vi "decode-from-json-cDAQ.vi"(8 "sensor-options-json":string, 10 "data-logging-json":string, 11 "filepath-json":string) -> (0 "Sensor Option Recall":T1={"Display Units"="log", "Zero Offset"=2.62, "Sensor Min"=0.0, "Sensor Max"=500.0, "Signal Min"=0.0, "Signal Max"=100.0, "Conversion Factor"=0.0}, 2 "Datalogging Recall":T2={"data-precision"=3, "Include Date"=FALSE, "Include Timestamp"=TRUE, "Include Milliseconds"=FALSE, "sample-rate (Hz)"=4.0, "Logging Active"=TRUE}, 3 "Filepath Recall":T3={"Log Filepath Source"=enum."Application Relative (Auto)", "Log File Path (Manual)"=path "C:/Users/dheard/Documents/0002-labview-projects/ammonia-absorbsion-rig/data", "Log File Folder Name"="data", "log file name"="log", "Include Date in Filename"=TRUE, "Include Time in Filename"=TRUE})   [LabVIEW 2024]
uses:
  utils-sub-vi/csv-file-logging-util/filepath-selection.ctl
  utils-sub-vi/csv-file-logging-util/datalogging-options.ctl
  sensor-options.ctl
  filepath-json-cluster-feck.ctl
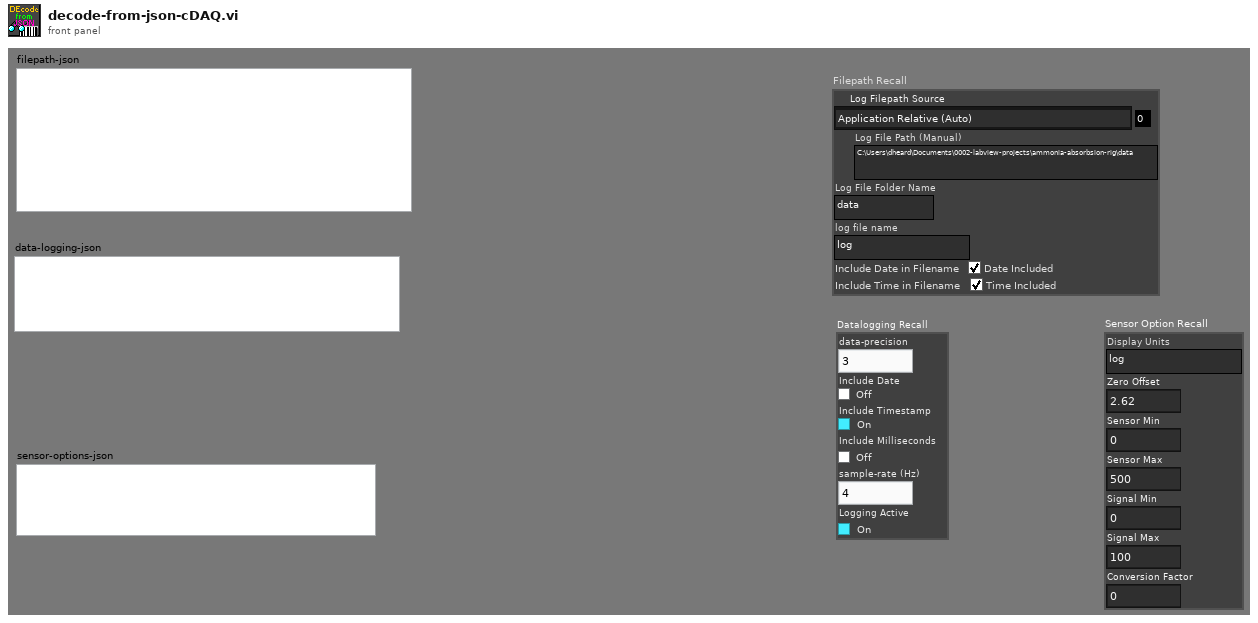
[diagram p1: front panel]
types:
  T1 = typedef "sensor-options.ctl" = cluster{"Display Units":string, "Zero Offset":dbl, "Sensor Min":dbl, "Sensor Max":dbl, "Signal Min":dbl, "Signal Max":dbl, "Conversion Factor":dbl}
  T2 = typedef "datalogging-options.ctl" = cluster{"data-precision":i32, "Include Date":bool, "Include Timestamp":bool, "Include Milliseconds":bool, "sample-rate (Hz)":dbl, "Logging Active":bool}
  T3 = typedef "filepath-selection.ctl" = cluster{"Log Filepath Source":enum16{"Application Relative (Auto)", "VI Relative (Auto)", "Complete Path (Manual)"}, "Log File Path (Manual)":path, "Log File Folder Name":string, "log file name":string, "Include Date in Filename":bool, "Include Time in Filename":bool}
  T4 = typedef "filepath-json-cluster-feck.ctl" = cluster{"Log Filepath Source":i32, "Log Filepath byte array":u8[], "Log File Folder Name":string, "log file name":string, "Include Date in Filename":bool, "Include Time in Filename":bool}
  T5 = enum16{"Application Relative (Auto)", "VI Relative (Auto)", "Complete Path (Manual)"}
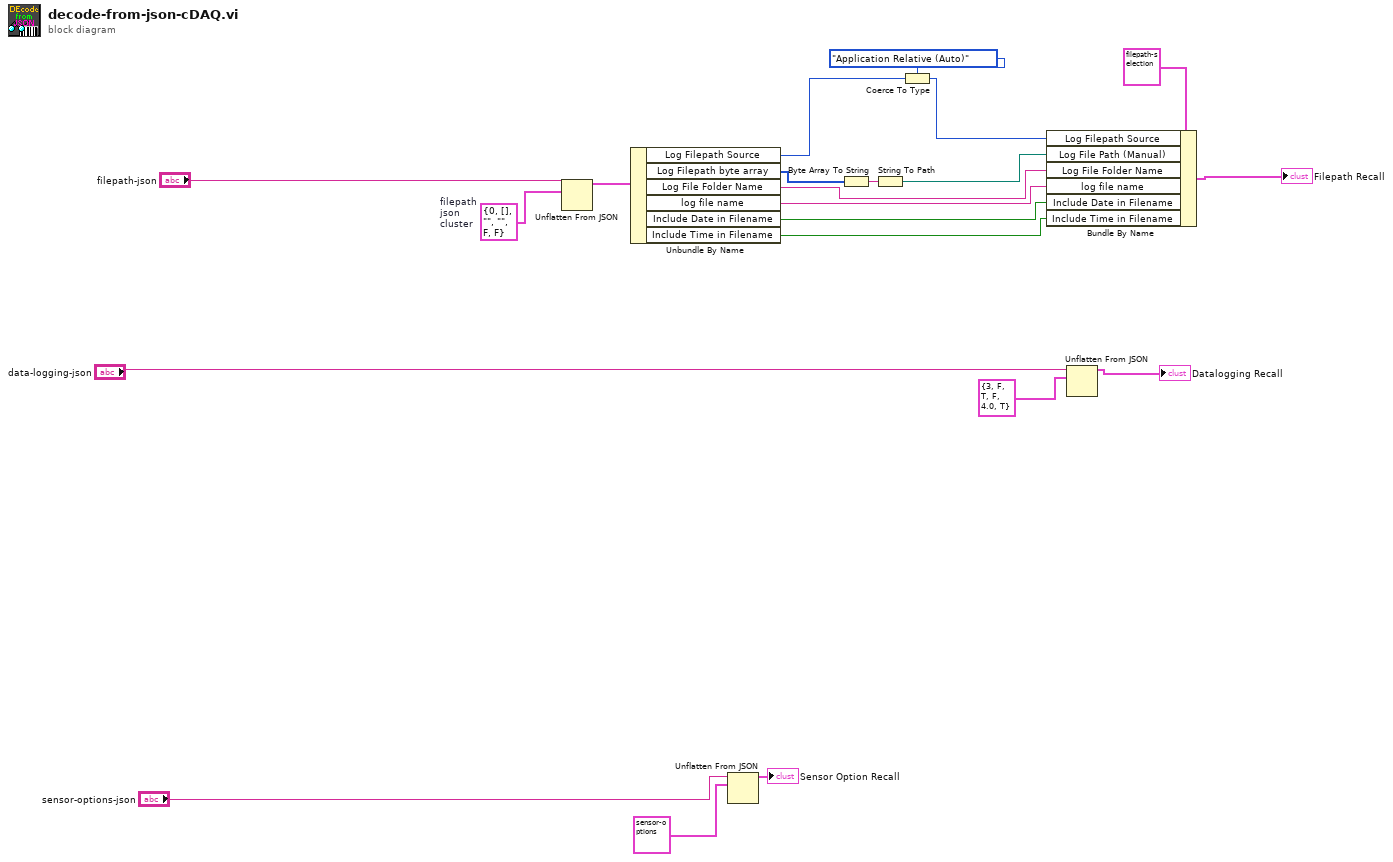
[diagram p0: block diagram]
diagram:
  w7 = T4 {"Log Filepath Source"=0, "Log Filepath byte array"=[], "Log File Folder Name"="", "log file name"="", "Include Date in Filename"=FALSE, "Include Time in Filename"=FALSE}  # filepath json cluster
  n1 = Unflatten From JSON(JSON string="filepath-json", type and defaults=w7) -> (value=w17:T4)  [unwired: 5 in, 1 out]
  n2 = Unbundle By Name(w17) -> ("Log Filepath Source"=w8:i32, "Log Filepath byte array"=w15:u8[], "Log File Folder Name"=w12:string, "log file name"=w11:string, "Include Date in Filename"=w10:bool, "Include Time in Filename"=w9:bool)
  n3 = Unflatten From JSON(JSON string="sensor-options-json", type and defaults=T1 {"Display Units"="units", "Zero Offset"=2.62, "Sensor Min"=0.0, "Sensor Max"=500.0, "Signal Min"=0.0, "Signal Max"=100.0, "Conversion Factor"=0.0} ("Sensor Options")) -> (value=→"Sensor Option Recall":T1)  [unwired: 5 in, 1 out]
  n4 = Byte Array To String(unsigned byte array=w15) -> (string=w14:string)
  n5 = String To Path(string=w14) -> (path=w13:path)
  n6 = Coerce To Type(0:w8, 1:T5."Application Relative (Auto)" ("Log Filepath Source")) -> (2:w19:T5)
  n7 = Bundle By Name(cluster=T3 {"Log Filepath Source"=enum."VI Relative (Auto)", "Log File Path (Manual)"=path "C:/Users/dheard/Documents/0002-labview-projects/ammonia-absorbsion-rig/data", "Log File Folder Name"="data", "log file name"="log", "Include Date in Filename"=TRUE, "Include Time in Filename"=TRUE} ("Filepath Selection"), "Log Filepath Source"=w19, "Log File Path (Manual)"=w13, "Log File Folder Name"=w12, "log file name"=w11, "Include Date in Filename"=w10, "Include Time in Filename"=w9) -> (→"Filepath Recall":T3)
  n8 = Unflatten From JSON(JSON string="data-logging-json", type and defaults=T2 {"data-precision"=3, "Include Date"=FALSE, "Include Timestamp"=TRUE, "Include Milliseconds"=FALSE, "sample-rate (Hz)"=4.0, "Logging Active"=TRUE} ("Datalogging options")) -> (value=→"Datalogging Recall":T2)  [unwired: 5 in, 1 out]
